vi "ResultUserEvent.vi"(8 "error in":errorcluster caption="错误输入（无错误）", 10 "Value":variant, 11 "Step":string) -> (0 "error out":errorcluster caption="错误输出")   [LabVIEW 2013]
uses:
  Ctl/ResultCtl.ctl
  Global.vi
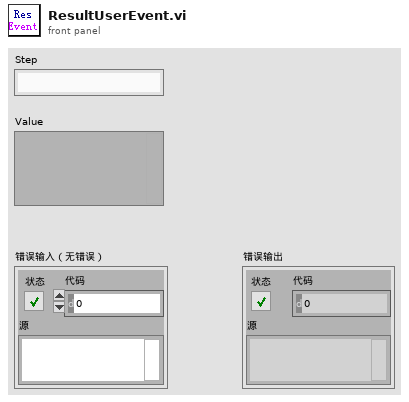
[diagram p1: front panel]
types:
  T1 = typedef "ResultCtl.ctl" = cluster{"Step":string, "Value":variant}
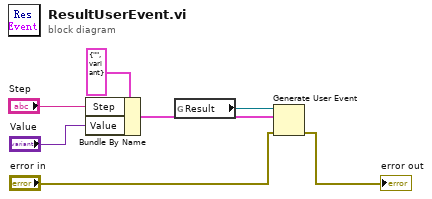
[diagram p0: block diagram]
diagram:
  n1 = Bundle By Name(cluster=T1 {"Step"="", "Value"=variant} ("Result"), "Step"="Step", "Value"="Value") -> (w5:T1)
  n2 = global read "Global.vi" "Result"() -> (w6:refnum<user-event>)
  n3 = Generate User Event(user event=w6, event data cluster=w5, error in="error in") -> (error out=→"error out":errorcluster)  [unwired: 1 in, 1 out]
